vi "反馈节点.vi"() -> ()   [LabVIEW 2020]
doc: "本VI是为《我和LabVIEW》一书编写的示例。\n关于本书的介绍请参考网页：\nhttp://ruanqizhen.spaces.live.com/blog/cns!5852D4F797C53FB6!4310.entry"
panel:
  out "result":dbl
  out "数值":dbl
  out "x+y":i32
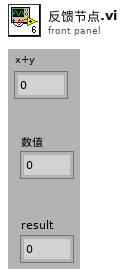
[diagram p1: front panel]
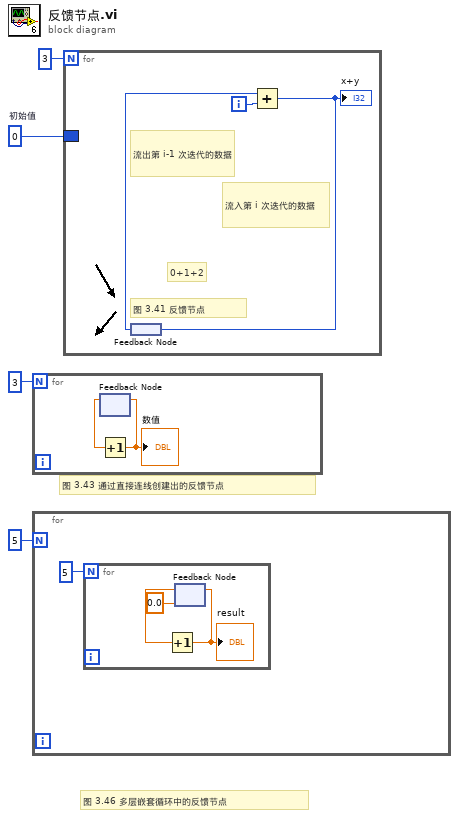
[diagram p0: block diagram]
diagram:
  w3 = 0  # 初始值
  # "图 3.46 多层嵌套循环中的反馈节点"
  # "图 3.43 通过直接连线创建出的反馈节点"
  n1 = for {
    N: 3 -> [_]
    n2 = feedback #1() -> (w6:dbl)  [unwired: 1 out]
    n3 = Increment(x=w6) -> (x+1=w5:dbl)
    "数值" <- w5
    n4 = feedback-in #1(w5) -> ()
  }
  n5 = for {
    N: 5 -> [_]
    n6 = for {
      N: 5 -> [_]
      n7 = feedback #2(0.0) -> (w10:dbl)
      n8 = Increment(x=w10) -> (x+1=w9:dbl)
      "result" <- w9
      n9 = feedback-in #2(w9) -> ()
    }
  }
  n10 = for {
    N: 3 -> [_]
    border: w3 -> [_]
    i -> [w11]
    # "图 3.41 反馈节点"
    # "0+1+2"
    # "流出第 i-1 次迭代的数据"
    # "流入第 i 次迭代的数据"
    n11 = feedback #3() -> (w12:i32)
    n12 = Add(x=w12, y=w11) -> (x+y=w13:i32)
    "x+y" <- w13
    n13 = feedback-in #3(w13) -> ()
  }
